vi "Control - PID Control.vi"() -> ()   [LabVIEW 2013, in "Control Workspace Object.lvlib"]
doc: "Sample numeric display item."
uses:
  Control Workspace Object.lvlib
  <vilib>/NI Veristand/Display Template Support/Display Template Support.llb/cluster_Screen Item Settings.ctl
  <vilib>/NI Veristand/Display Template Support/Display Template Support.llb/cluster_Graph Scale Settings.ctl
  <vilib>/NI Veristand/Display Template Support/Display Template Support.llb/cluster_Graph Plot Settings.ctl
  NationalInstruments.VeriStand.SystemStorage
  <vilib>/NI Veristand/Display Template Support/Display Template Support.llb/enum_Display Template Handler Minimal To Widget Msg.ctl
  <vilib>/NI Veristand/Display Template Support/Display Template Support.llb/enum_Display Template Handler Minimal To Workspace.ctl
  Shared/Types/Workspace Object State Variables.ctl
  Types/UI.Refs.ctl
  Shared/Types/UDP Streaming Command Cluster.ctl
  Shared/Types/UDP Streaming State.ctl
  Shared/Types/Workspace Object Cached Settings.ctl
  <vilib>/NI Veristand/Execution/Workspace/WorkspaceAPI.ctl
  <vilib>/NI Veristand/Execution/Workspace/SystemStateRegEventRef.ctl
  <vilib>/NI Veristand/Execution/Workspace/SystemStateEventRef.ctl
  <vilib>/NI Veristand/Display Template Support/Display Template Support.llb/sub_Display Template Handler Custom.vi
  Shared/Constants.vi
  <vilib>/NI Veristand/Execution/Workspace/NI VeriStand - Get Multiple Channel Values.vi
  <vilib>/NI Veristand/Execution/Workspace/NI VeriStand - Set Single Channel Value.vi
  Shared/Control Addon Shared.lvlib
  <vilib>/NI Veristand/Execution/Workspace/NI_VS Workspace ExecutionAPI.lvlib
  NationalInstruments.VeriStand.ClientAPI
panel:
  in  "Manual Value":bool
  in  "Revert":bool
  in  "Apply":bool
  in  "Manual Output":dbl
  in  "Manual Control":bool
  in  "Setpoint":dbl
  in  "NIVS.System Definition Root":refnum<k24>
  in  "NIVS.Gateway IP Address":string
  in  "T = PID":bool=TRUE
  in  "Hold":bool
  in  "Autoscale Y":bool=TRUE
  in  "Autoscale X":bool=TRUE
  out "Chart":waveform(dbl)[](graph)
  out "Control Name":string
  in  "Item.Data":T1
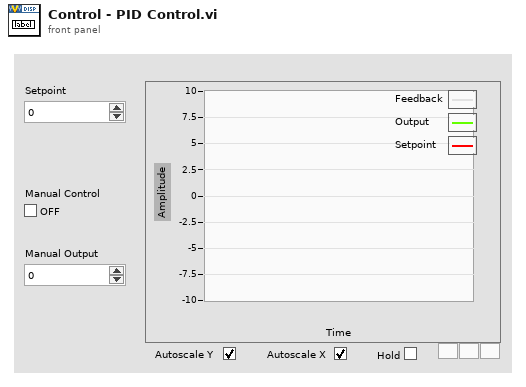
[diagram p1: front panel]
types:
  T1 = typedef "cluster_Screen Item Settings.ctl" = cluster{"Template VI":string, "Position X":i32, "Position Y":i32, "Custom":string, "Show Title Bar":bool, "ID":i32, "Always On Top":bool, "Allow Resize":bool, "Allow Minimize":bool, "Allow Close":bool, "Size to Screen":bool, "Screen.ID":i32, "State":enum16{"Normal", "New"}, "Title":string, "Window Bounds":cluster{"[0]":i16, "[1]":i16, "[2]":i16, "[3]":i16}, "Channel Ref":u64, "Unit":string, "Default Units?":bool, "Flash Limit?":bool, "Color 1":u32, "Color 2":u32, "Color 3":u32, "Color 4":u32, "Bck Color":u32, "Fore Color":u32, "Limit 1":dbl, "Limit 2":dbl, "Limit 3":dbl, "Limit 4":dbl, "Limit Mode 1":i32, "Limit Mode 2":i32, "Limit Mode 3":i32, "Limit Mode 4":i32, "Scale Precision":i32, "Scale Min":dbl, "Scale Max":dbl, "Format":i32, "Precision":i32, "Background Type":i32, "IDs":i32[], "Units":string[], "Labels":string[], "Scale Factor":dbl, "Scale Offset":dbl, "YScale Index":u32[], "XScale":T2, "YScales":T2[], "Plots":T3[], "Update Period":dbl, "History Length":dbl, "My.Ref":refnum<vi>, "Is Control?":bool, "Channel Paths":string[], "Custom Data":variant}
  T2 = typedef "cluster_Graph Scale Settings.ctl" = cluster{"Format":u8, "Precision":u8, "Fit":u8, "Label":string, "Use Default Label":bool, "Label Visible":bool, "Min":dbl, "Max":dbl}
  T3 = typedef "cluster_Graph Plot Settings.ctl" = cluster{"Bar Style":u8, "Fill To":i16, "Fill/PtColor":u32, "Line Style":u8, "Line Width":u8, "Color":u32, "Interp":u8, "Point Style":u8}
  T4 = typedef "Control Addon Shared.lvlib/Workspace Object State Variables.ctl" = cluster{"UI.Refs":T5, "Addon.GUID":string, "Addon.Name":string, "Addon.Type":enum16{"PID", "Industrial"}, "Data.UDPEngineQueue":refnum<queue>, "Data.Found?":bool, "Data.UDPChannels":string[], "Data.PreviousValues":dbl[], "Data.SlowChannels":string[], "Data.PendingChange?":bool, "CachedData.UserEvent":refnum<user-event>, "CachedData.Data":T6, "Workspace.Connected?":bool, "NIVS.SysDef":refnum<k24>, "NIVS.WorkspaceManager":T7, "NIVS.UserEventRefs":cluster{"Event Registration Refnum":refnum<event-registration>, "SystemChangeEventRef":T8}, "NIVS.SystemStateRefs":T9, "NIVS.LaunchRef":refnum<user-event>}
  T5 = typedef "Control Addon Shared.lvlib/UI.Refs.ctl" = cluster{"Chart":refnum<vi>, "Manual Value":refnum<vi>, "Manual Output":refnum<vi>, "Revert":refnum<vi>, "Apply":refnum<vi>}
  T6 = typedef "Control Addon Shared.lvlib/Workspace Object Cached Settings.ctl" = cluster{"Path":string}
  T7 = typedef "NI_VS Workspace ExecutionAPI.lvlib/WorkspaceAPI.ctl" = refnum<k24>
  T8 = typedef "NI_VS Workspace ExecutionAPI.lvlib/SystemStateRegEventRef.ctl" = refnum<event-registration>
  T9 = typedef "NI_VS Workspace ExecutionAPI.lvlib/SystemStateEventRef.ctl" = cluster{"CustDatRef":refnum<user-event>, "EvtRef":refnum<k27>}
  T10 = typedef "enum_Display Template Handler Minimal To Workspace.ctl" = cluster{"Operation":enum16{"SetCustomData", "DeleteItem"}, "Data":variant}
  T11 = typedef "enum_Display Template Handler Minimal To Widget Msg.ctl" = enum16{"Stop", "LaunchConfigDialog"}
  T12 = typedef "Control Addon Shared.lvlib/UDP Streaming Command Cluster.ctl" = cluster{"Action":T13, "Channels":string[]}
  T13 = typedef "Control Addon Shared.lvlib/UDP Streaming State.ctl" = enum8{"Idle", "Start Acq", "Run", "Stop Acq", "Exit"}
  T14 = cluster{"Event Registration Refnum":refnum<event-registration>, "SystemChangeEventRef":T8}
  T15 = typedef "NI_VS Workspace ExecutionAPI.lvlib/SystemState.ctl" = u8
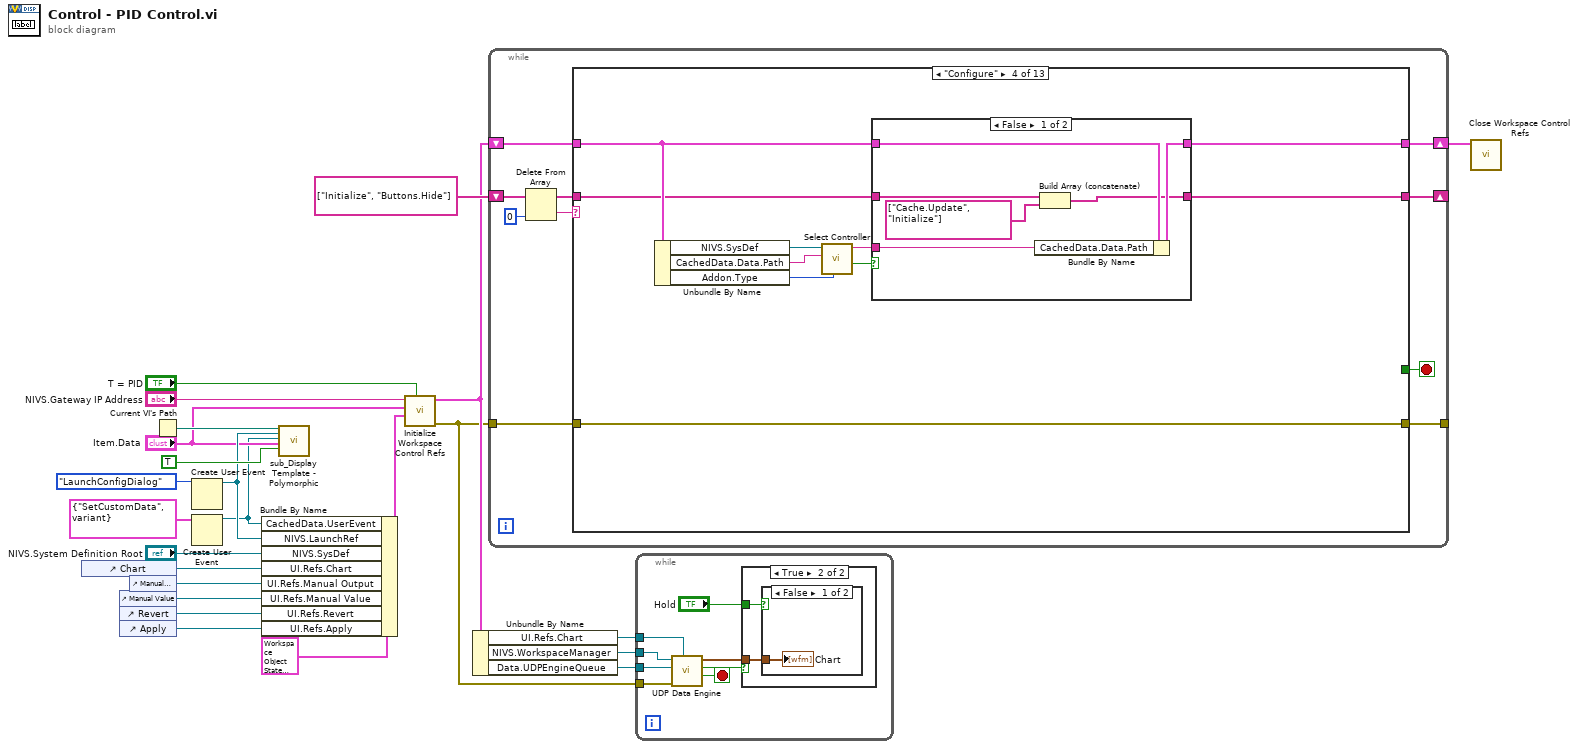
[diagram p0: block diagram]
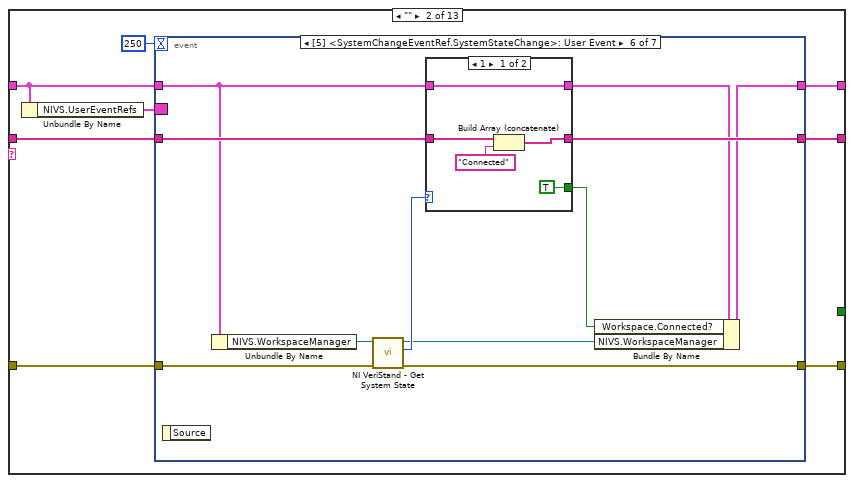
[diagram p5: hidden frame]
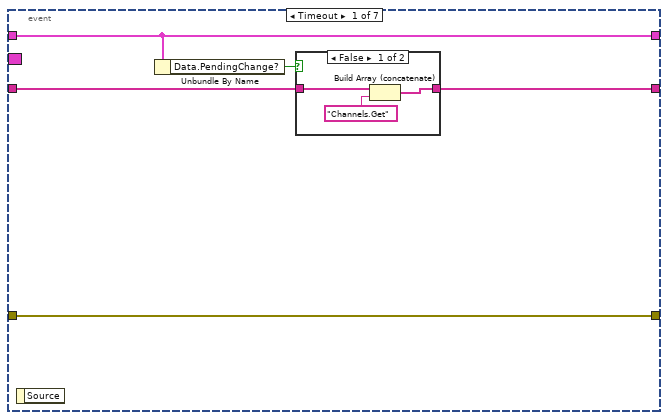
[diagram p6: hidden frame]
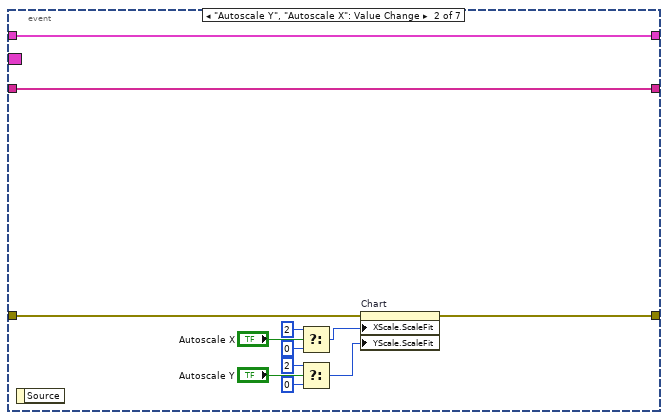
[diagram p8: hidden frame]
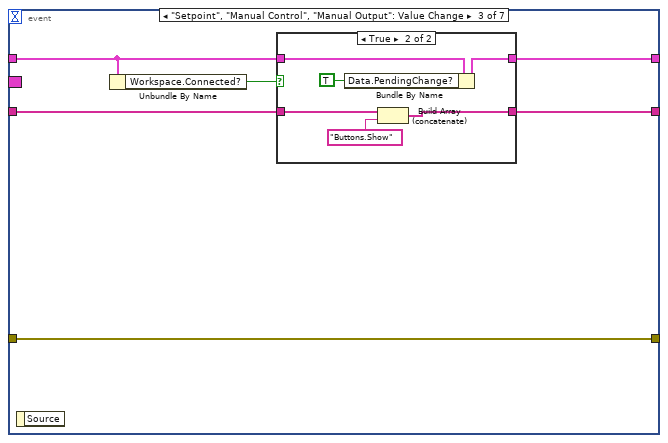
[diagram p9: hidden frame]
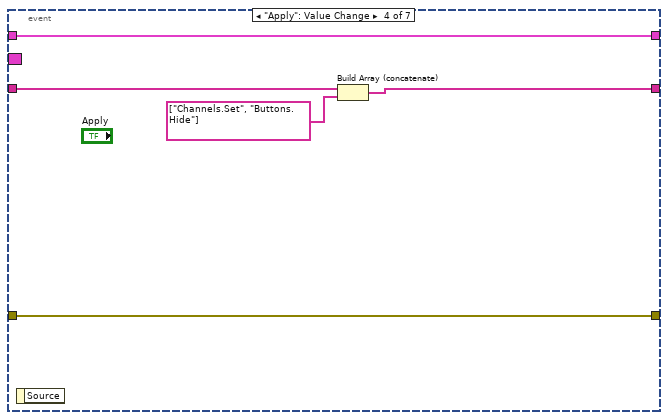
[diagram p11: hidden frame]
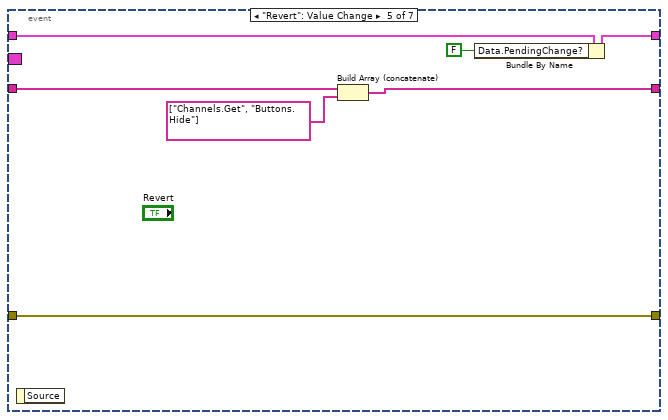
[diagram p12: hidden frame]
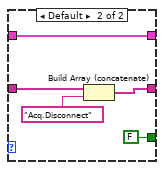
[diagram p13: hidden frame]
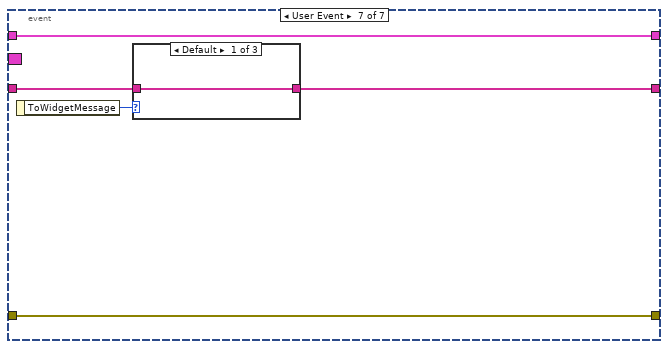
[diagram p14: hidden frame]
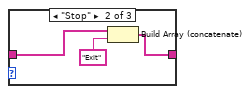
[diagram p15: hidden frame]
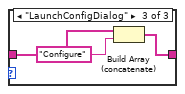
[diagram p16: hidden frame]
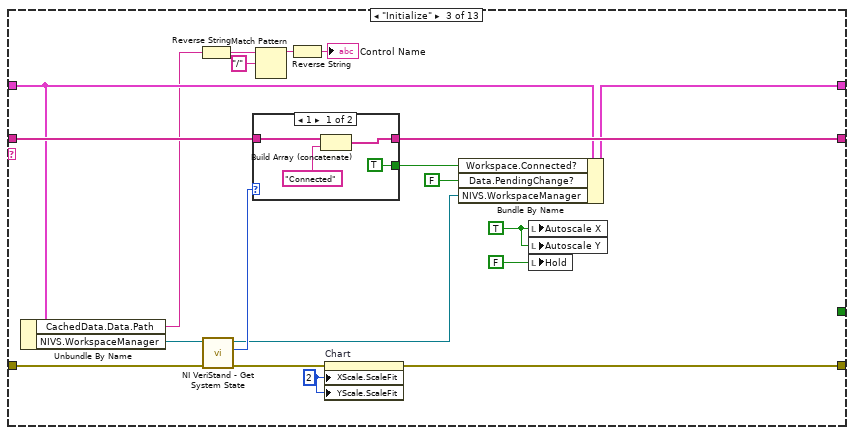
[diagram p17: hidden frame]
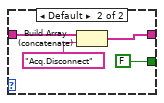
[diagram p18: hidden frame]
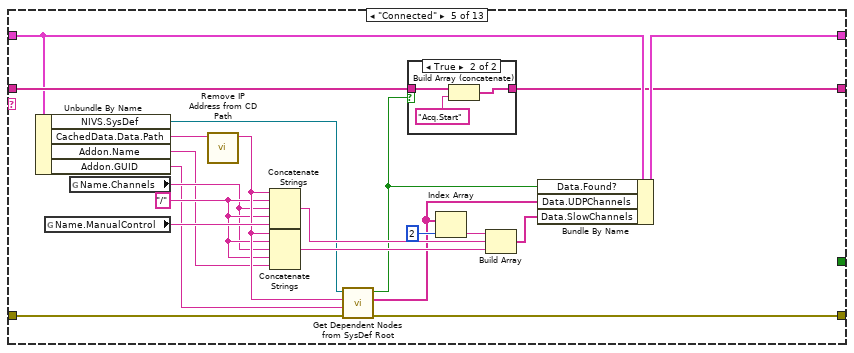
[diagram p20: hidden frame]
diagram:
  n1 = control-ref of="Chart"() -> (w12:refnum<vi>)
  n2 = control-ref of="Manual Value"() -> (w10:refnum<vi>)
  n3 = control-ref of="Revert"() -> (w9:refnum<vi>)
  n4 = control-ref of="Apply"() -> (w8:refnum<vi>)
  n5 = control-ref of="Manual Output"() -> (w11:refnum<vi>)
  n6 = Current VI's Path() -> (path=w22:path)
  n7 = Create User Event(user event datatype=enum_Display_Template_Handler_Minimal_To_Widget_Msg."LaunchConfigDialog" ("ToWidgetMessage")) -> (user event=w7:refnum<user-event>)  [unwired: 1 in, 1 out]
  n8 = Create User Event(user event datatype=T10 {"Operation"=enum."SetCustomData", "Data"=variant} ("Data")) -> (user event=w2:refnum<user-event>)  [unwired: 1 in, 1 out]
  n9 = Bundle By Name(cluster=T4 {"UI.Refs"={"Chart"=refnum, "Manual Value"=refnum, "Manual Output"=refnum, "Revert"=refnum, "Apply"=refnum}, "Addon.GUID"="", "Addon.Name"="", "Addon.Type"=enum."PID", "Data.UDPEngineQueue"=refnum, "Data.Found?"=FALSE, "Data.UDPChannels"=[], "Data.PreviousValues"=[], "Data.SlowChannels"=[], "Data.PendingChange?"=FALSE, "CachedData.UserEvent"=refnum, "CachedData.Data"={"Path"=""}, "Workspace.Connected?"=FALSE, "NIVS.SysDef"=refnum, "NIVS.WorkspaceManager"=refnum, "NIVS.UserEventRefs"={"Event Registration Refnum"=refnum, "SystemChangeEventRef"=refnum}, "NIVS.SystemStateRefs"={"CustDatRef"=refnum, "EvtRef"=refnum}, "NIVS.LaunchRef"=refnum}, "CachedData.UserEvent"=w2, "NIVS.LaunchRef"=w7, "NIVS.SysDef"="NIVS.System Definition Root", "UI.Refs.Chart"=w12, "UI.Refs.Manual Output"=w11, "UI.Refs.Manual Value"=w10, "UI.Refs.Revert"=w9, "UI.Refs.Apply"=w8) -> (w4:T4)
  n10 = call-poly <vilib>:"sub_Display Template - Polymorphic.vi"("Parent.Path"=w22, "ToWidgetEvent"=w7, "ToWorkspace"=w2, "Item.Data"="Item.Data", "Resizable"=TRUE) -> ()  [unwired: 1 in, 14 out]
  n11 = call "Initialize Workspace Control Refs.vi"("T = PID"="T = PID", "State Variables in"=w4, "Item.Data"="Item.Data", "NIVS.Gateway IP Address"="NIVS.Gateway IP Address") -> ("error out"=w1:errorcluster, "State Variables out"=w15:T4)  [unwired: 6 in]
  n12 = Unbundle By Name(w15) -> ("UI.Refs.Chart"=w17:refnum<vi>, "NIVS.WorkspaceManager"=w16:T7, "Data.UDPEngineQueue"=w14:refnum<queue>)
  n13 = while {
    shift-right: [w28] -> _
    shift-left: string[] ["Initialize", "Buttons.Hide"] -> [w32]
    tunnel: w1 -> [w30]
    tunnel: [w27] -> _
    shift-right: [w26] -> w19
    shift-left: w15 -> [w25]
    stop <- w34 stop-if-true
    n14 = Delete From Array(array=w32, index=0) -> (deleted portion=w31:string, array with subset deleted=w29:string[])  [unwired: 1 in]
    n15 = case shown="\"Configure\"" w31 {
      tunnel: [_ _ _ _ _ TRUE _ _ _ _ _ _ _] -> w34
      tunnel: [w37 w44 w142 w157 w181 w206 w213 w221 w229 w235 w241 w252 w304] -> w28
      tunnel: w30 -> [w36 w42 w144 w163 w173 w201 w212 w216 w228 w231 w237 w249 w292]
      tunnel: w29 -> [w37 w43 w143 w156 w192 w206 w213 w221 w229 w235 w241 w252 w304]
      tunnel: w25 -> [w35 w38 w130 w161 w190 w198 w209 w220 w224 w234 w240 w242 w290]
      tunnel: [w36 w41 w126 w163 w191 w200 w212 w215 w227 w230 w236 w248 w291] -> w27
      tunnel: [w35 w40 w137 w160 w189 w198 w209 w220 w224 w234 w240 w247 w289] -> w26
      frame Default {
      }
      frame "" {
        n16 = Unbundle By Name(w38) -> ("NIVS.UserEventRefs"=w39:T14)
        n17 = event shown="[5] <SystemChangeEventRef.SystemStateChange>: User Event" {
          selector: w39 -> [_ _ _ _ _ _ _]
          dyn-events: _ -> [_ _ _ _ _ _ _]
          timeout: 250 -> [_ _ _ _ _ _ _]
          tunnel: [w48 w66 w69 w81 w89 w99 w117] -> w44
          tunnel: w43 -> [w49 w66 w70 w82 w90 w100 w116]
          tunnel: w42 -> [w50 w60 w72 w85 w92 w103 w115]
          tunnel: [w50 w59 w72 w85 w92 w102 w115] -> w41
          tunnel: [w47 w65 w71 w84 w87 w98 w114] -> w40
          tunnel: w38 -> [w47 w65 w68 w84 w88 w95 w114]
          event Timeout {
            n18 = event-data() -> ()  [unwired: 2 out]
            n19 = Unbundle By Name(w47) -> ("Data.PendingChange?"=w46:bool)
            n20 = case shown="False" w46 {
              tunnel: w49 -> [w52 w54]
              tunnel: [w51 w54] -> w48
              frame False {
                n21 = Build Array (concatenate)(w52, "Channels.Get") -> (w51:string[])
              }
              frame True {
              }
            }
          }
          event "Autoscale Y", "Autoscale X": Value Change {
            n22 = event-data() -> ()  [unwired: 2 out]
            n23 = Select(t=u8 2, s="Autoscale X", f=u8 0 ("X Scale.Scale Fit")) -> (s? t:f=w62:u8)
            n24 = Select(t=u8 2, s="Autoscale Y", f=u8 0 ("X Scale.Scale Fit")) -> (s? t:f=w55:u8)
            n25 = property on="Chart" class="WFChart (strict)"(error in=w60, "XScale.ScaleFit"=w62, "YScale.ScaleFit"=w55) -> (error out=w59:errorcluster)  [unwired: 1 in, 1 out]
          }
          event "Setpoint", "Manual Control", "Manual Output": Value Change {
            n26 = event-data() -> ()  [unwired: 2 out]
            n27 = Unbundle By Name(w68) -> ("Workspace.Connected?"=w67:bool)
            n28 = case shown="True" w67 {
              tunnel: w68 -> [w73 w79]
              tunnel: [w73 w78] -> w71
              tunnel: w70 -> [w74 w77]
              tunnel: [w74 w75] -> w69
              frame False {
              }
              frame True {
                n29 = Bundle By Name(cluster=w79, "Data.PendingChange?"=TRUE ("Pending Change?")) -> (w78:T4)
                n30 = Build Array (concatenate)(w77, "Buttons.Show") -> (w75:string[])
              }
            }
          }
          event "Apply": Value Change {
            n31 = event-data() -> ()  [unwired: 2 out]
            n32 = Build Array (concatenate)(w82, string[] ["Channels.Set", "Buttons.Hide"]) -> (w81:string[])
          }
          event "Revert": Value Change {
            n33 = event-data() -> ()  [unwired: 2 out]
            n34 = Build Array (concatenate)(w90, string[] ["Channels.Get", "Buttons.Hide"]) -> (w89:string[])
            n35 = Bundle By Name(cluster=w88, "Data.PendingChange?"=FALSE ("Pending Change?")) -> (w87:T4)
          }
          event User Event {
            n36 = event-data() -> ()  [unwired: 2 out]
            n37 = Unbundle By Name(w95) -> ("NIVS.WorkspaceManager"=w94:T7)
            n38 = call <vilib>:"NI VeriStand - Get System State.vi"("error in (no error)"=w103, "WorkspaceManager in"=w94) -> ("error out"=w102:errorcluster, "System State"=w101:T15, "WorkspaceManager  out"=w93:T7)  [unwired: 5 in, 2 out]
            n39 = case shown="1" w101 {
              tunnel: w100 -> [w108 w113]
              tunnel: [w107 w112] -> w99
              tunnel: [w105 w110] -> w97
              tunnel: w95 -> [w105 w110]
              tunnel: [TRUE FALSE] -> w96
              frame 1 {
                n40 = Build Array (concatenate)(w108, "Connected") -> (w107:string[])
              }
              frame Default {
                n41 = Build Array (concatenate)(w113, "Acq.Disconnect") -> (w112:string[])
              }
            }
            n42 = Bundle By Name(cluster=w97, "Workspace.Connected?"=w96, "NIVS.WorkspaceManager"=w93) -> (w98:T4)
          }
          event User Event {
            n43 = event-data() -> ("ToWidgetMessage"=w118:T11)  [unwired: 1 out]
            n44 = case shown="Default" w118 {
              tunnel: [w119 w121 w124] -> w117
              tunnel: w116 -> [w119 w122 w125]
              frame Default {
              }
              frame "Stop" {
                n45 = Build Array (concatenate)(w122, "Exit") -> (w121:string[])
              }
              frame "LaunchConfigDialog" {
                n46 = Build Array (concatenate)(w125, "Configure") -> (w124:string[])
              }
            }
          }
        }
      }
      frame "Initialize" {
        w134 = u8 2 ("X Scale.Scale Fit")
        w135 = TRUE ("Autoscale X")
        n47 = Unbundle By Name(w130) -> ("CachedData.Data.Path"=w128:string, "NIVS.WorkspaceManager"=w129:T7)
        n48 = Reverse String(1:w128) -> (0:w141:string)
        n49 = call <vilib>:"NI VeriStand - Get System State.vi"("error in (no error)"=w144, "WorkspaceManager in"=w129) -> ("error out"=w133:errorcluster, "System State"=w145:T15, "WorkspaceManager  out"=w127:T7)  [unwired: 5 in, 2 out]
        n50 = case shown="1" w145 {
          tunnel: w143 -> [w149 w153]
          tunnel: [w148 w152] -> w142
          tunnel: [TRUE FALSE] -> w136
          frame 1 {
            n51 = Build Array (concatenate)(w149, "Connected") -> (w148:string[])
          }
          frame Default {
            n52 = Build Array (concatenate)(w153, "Acq.Disconnect") -> (w152:string[])
          }
        }
        n53 = Match Pattern(string=w141, regular expression="/") -> (before substring=w138:string)  [unwired: 1 in, 3 out]
        n54 = Reverse String(1:w138) -> (0:→"Control Name":string)
        n55 = property on="Chart" class="WFChart (strict)"(error in=w133, "XScale.ScaleFit"=w134, "YScale.ScaleFit"=w134) -> (error out=w126:errorcluster)  [unwired: 1 in, 1 out]
        n56 = Bundle By Name(cluster=w130, "Workspace.Connected?"=w136, "Data.PendingChange?"=FALSE ("Pending Change?"), "NIVS.WorkspaceManager"=w127) -> (w137:T4)
        n57 = local write "Autoscale X"(w135) -> ()
        n58 = local write "Autoscale Y"(w135) -> ()
        n59 = local write "Hold"(FALSE ("Hold")) -> ()
      }
      frame "Configure" {
        n60 = Unbundle By Name(w161) -> ("NIVS.SysDef"=w155:refnum<k24>, "CachedData.Data.Path"=w162:string, "Addon.Type"=w154:enum16{"PID", "Industrial"})
        n61 = call "Select Controller.vi"("Type"=w154, "CD Path"=w162, "NIVS.System Definition Root"=w155) -> ("Cancelled?"=w159:bool, "Custom Device Path Out"=w158:string)  [unwired: 6 in, 1 out]
        n62 = case shown="False" w159 {
          tunnel: w161 -> [w169 w170]
          tunnel: [w168 w170] -> w160
          tunnel: w158 -> [w167 _]
          tunnel: [w165 w171] -> w157
          tunnel: w156 -> [w166 w171]
          frame False {
            n63 = Bundle By Name(cluster=w169, "CachedData.Data.Path"=w167) -> (w168:T4)
            n64 = Build Array (concatenate)(w166, string[] ["Cache.Update", "Initialize"]) -> (w165:string[])
          }
          frame True {
          }
        }
      }
      frame "Connected" {
        w178 = "/" ("string")
        n65 = Unbundle By Name(w190) -> ("NIVS.SysDef"=w174:refnum<k24>, "CachedData.Data.Path"=w188:string, "Addon.Name"=w175:string, "Addon.GUID"=w172:string)
        n66 = global read "Constants.vi" "Name.ManualControl"() -> (w187:string)
        n67 = global read "Constants.vi" "Name.Channels"() -> (w177:string)
        n68 = call "Remove IP Address from CD Path.vi"("CD Path"=w188) -> ("Path"=w186:string)  [unwired: 10 in]
        n69 = Concatenate Strings(w186, w178, w177, w178, w187) -> (w185:string)
        n70 = Concatenate Strings(w186, w178, w177, w178, w175) -> (w184:string)
        n71 = call "Get Dependent Nodes from SysDef Root.vi"("error in (no error)"=w173, "GUID"=w172, "Path"=w186, "SysDef Ref"=w174) -> ("error out"=w191:errorcluster, "Channels"=w180:string[], "Found"=w176:bool)  [unwired: 5 in]
        n72 = case shown="True" w176 {
          tunnel: w192 -> [w193 w196]
          tunnel: [w193 w195] -> w181
          frame False {
          }
          frame True {
            n73 = Build Array (concatenate)(w196, "Acq.Start") -> (w195:string[])
          }
        }
        n74 = Index Array(array=w180, index=2) -> (element=w182:string)
        n75 = Build Array(w182, w185, w184) -> (w179:string[])
        n76 = Bundle By Name(cluster=w190, "Data.Found?"=w176, "Data.UDPChannels"=w180, "Data.SlowChannels"=w179) -> (w189:T4)
      }
      frame "Exit" {
        n77 = Unbundle By Name(w198) -> ("Data.UDPEngineQueue"=w197:refnum<queue>)
        n78 = Enqueue Element(queue=w197, element=T12 {"Action"=enum."Stop Acq", "Channels"=[]}, error in (no error)=w201) -> (queue out=w204:refnum<queue>, error out=w202:errorcluster)  [unwired: 1 in, 1 out]
        n79 = Enqueue Element(queue=w204, element=T12 {"Action"=enum."Exit", "Channels"=[]}, error in (no error)=w202) -> (error out=w200:errorcluster)  [unwired: 1 in, 2 out]
      }
      frame "Cache.Update" {
        n80 = Unbundle By Name(w209) -> ("CachedData.UserEvent"=w207:refnum<user-event>, "CachedData.Data"=w208:T6)
        n81 = Bundle By Name(cluster=T10 {"Operation"=enum."SetCustomData", "Data"=variant} ("event data"), "Data"=w208) -> (w210:T10)
        n82 = Generate User Event(user event=w207, event data cluster=w210) -> ()  [unwired: 2 in, 2 out]
      }
      frame "Acq.Start" {
        n83 = Unbundle By Name(w220) -> ("Data.UDPEngineQueue"=w214:refnum<queue>, "Data.UDPChannels"=w218:string[])
        n84 = Bundle By Name(cluster=T12 {"Action"=enum."Start Acq", "Channels"=[]}, "Channels"=w218) -> (w217:T12)
        n85 = Enqueue Element(queue=w214, element=w217, error in (no error)=w216) -> (error out=w215:errorcluster)  [unwired: 1 in, 2 out]
      }
      frame "Acq.Disconnect" {
        w222 = FALSE ("Manual Control")
        w225 = 0.0 ("Setpoint")
        n86 = Unbundle By Name(w224) -> ("Data.UDPEngineQueue"=w223:refnum<queue>)
        n87 = Enqueue Element(queue=w223, element=T12 {"Action"=enum."Stop Acq", "Channels"=[]}, error in (no error)=w228) -> (error out=w227:errorcluster)  [unwired: 1 in, 2 out]
        n88 = local write "Setpoint"(w225) -> ()
        n89 = local write "Manual Output"(w225) -> ()
        n90 = local write "Manual Control"(w222) -> ()
        n91 = local write "Manual Value"(w222) -> ()
      }
      frame "Buttons.Hide" {
        w232 = FALSE ("Hold")
        n92 = property on="Apply" class="Bool"(error in=w231, "Visible"=w232) -> (error out=w233:errorcluster)  [unwired: 1 in, 1 out]
        n93 = property on="Revert" class="Bool"(error in=w233, "Visible"=w232) -> (error out=w230:errorcluster)  [unwired: 1 in, 1 out]
      }
      frame "Buttons.Show" {
        w238 = TRUE ("Hold")
        n94 = property on="Apply" class="Bool"(error in=w237, "Visible"=w238) -> (error out=w239:errorcluster)  [unwired: 1 in, 1 out]
        n95 = property on="Revert" class="Bool"(error in=w239, "Visible"=w238) -> (error out=w236:errorcluster)  [unwired: 1 in, 1 out]
      }
      frame "Channels.Get" {
        n96 = Unbundle By Name(w242) -> ("Data.PendingChange?"=w243:bool, "Addon.Type"=w246:enum16{"PID", "Industrial"}, "Data.Found?"=w250:bool, "Workspace.Connected?"=w251:bool, "NIVS.WorkspaceManager"=w245:T7, "Data.SlowChannels"=w244:string[])
        n97 = case shown="False" w243 {
          tunnel: w251 -> [w269 _]
          tunnel: w250 -> [w263 _]
          tunnel: w249 -> [w260 w283]
          tunnel: [w259 w283] -> w248
          tunnel: [w258 w284] -> w247
          tunnel: w246 -> [w257 _]
          tunnel: w245 -> [w256 _]
          tunnel: w244 -> [w254 _]
          tunnel: w242 -> [w253 w284]
          frame False {
            n98 = Compound Arithmetic op=AND(w263, w269) -> (w264:bool)
            n99 = case shown="True" w264 {
              tunnel: w260 -> [w276 w282]
              tunnel: [w276 w281] -> w259
              tunnel: w256 -> [w275 w280]
              tunnel: [w275 w279] -> w255
              tunnel: w254 -> [_ w278]
              tunnel: [dbl[] [0.0, 0.0, 0.0] ("Values") w277] -> w268
              frame False {
              }
              frame True {
                n100 = call-poly <vilib>:"NI VeriStand - Get Channel Value.vi"("error in (no error)"=w282, "Channels"=w278, "WorkspaceManager in"=w280) -> ("error out"=w281:errorcluster, "Values"=w277:dbl[], "WorkspaceManager out"=w279:T7)  [unwired: 6 in]
              }
            }
            n101 = Index Array(array=w268) -> (element #1=w267:dbl, element #2=w262:dbl, element #3=w261:dbl)  [unwired: 3 in]
            n102 = To Long Integer(number=w262) -> (32bit integer=w266:i32)
            n103 = case shown="\"Industrial\"" w257 {
              tunnel: w261 -> [w271 w273]
              frame "Industrial" {
                n104 = To Long Integer(number=w271) -> (32bit integer=w272:i32)
                n105 = Not Equal To 0?(x=w272) -> (x != 0?=w270:bool)
                n106 = local write "Manual Value"(w270) -> ()
              }
              frame "PID" {
                n107 = local write "Manual Output"(w273) -> ()
              }
            }
            n108 = Not Equal To 0?(x=w266) -> (x != 0?=w265:bool)
            n109 = local write "Setpoint"(w267) -> ()
            n110 = local write "Manual Control"(w265) -> ()
            n111 = Bundle By Name(cluster=w253, "NIVS.WorkspaceManager"=w255, "Data.PreviousValues"=w268) -> (w258:T4)
          }
          frame True {
          }
        }
      }
      frame "Channels.Set" {
        n112 = Unbundle By Name(w290) -> ("Data.Found?"=w295:bool, "Workspace.Connected?"=w298:bool, "Data.PreviousValues"=w297:dbl[], "Data.SlowChannels"=w299:string[], "NIVS.WorkspaceManager"=w287:T7, "Addon.Type"=w285:enum16{"PID", "Industrial"})
        n113 = case shown="\"Industrial\"" w285 {
          tunnel: [w306 "Manual Output"] -> w293
          frame "Industrial" {
            n114 = Boolean To (0,1)(Boolean="Manual Value") -> (0, 1=w306:i16)
          }
          frame "PID" {
          }
        }
        n115 = Boolean To (0,1)(Boolean="Manual Control") -> (0, 1=w294:i16)
        n116 = Build Array("Setpoint", w294, w293) -> (w300:dbl[])
        n117 = Not Equal?(x=w297, y=w300) -> (x != y?=w303:bool[])
        n118 = Compound Arithmetic op=AND(w295, w298) -> (w296:bool)
        n119 = case shown="True" w296 {
          tunnel: w303 -> [_ w316]
          tunnel: w300 -> [_ w315]
          tunnel: w292 -> [w309 w314]
          tunnel: [w309 w313] -> w291
          tunnel: w287 -> [w308 w312]
          tunnel: [w308 w311] -> w286
          tunnel: w299 -> [_ w310]
          frame False {
          }
          frame True {
            n120 = for {
              shift-right: [w322] -> w313
              shift-left: w314 -> [w323]
              shift-right: [w321] -> w311
              shift-left: w312 -> [w320]
              tunnel: w316 -> [w319] mode=indexing
              tunnel: w315 -> [w318] mode=indexing
              tunnel: w310 -> [w317] mode=indexing
              n121 = case shown="True" w319 {
                tunnel: w323 -> [w325 w331]
                tunnel: [w325 w330] -> w322
                tunnel: [w324 w329] -> w321
                tunnel: w320 -> [w324 w328]
                tunnel: w318 -> [_ w327]
                tunnel: w317 -> [_ w326]
                frame False {
                }
                frame True {
                  n122 = call-poly <vilib>:"NI VeriStand - Set Channel Value.vi"("error in (no error)"=w331, "Value"=w327, "Channel"=w326, "WorkspaceManager in"=w328) -> ("error out"=w330:errorcluster, "WorkspaceManager out"=w329:T7)  [unwired: 6 in]
                }
              }
            }
          }
        }
        n123 = Bundle By Name(cluster=w290, "Data.PendingChange?"=FALSE ("Pending Change?"), "NIVS.WorkspaceManager"=w286) -> (w289:T4)
      }
    }
  }
  n124 = while {
    tunnel: w16 -> [w334]
    tunnel: w14 -> [w339]
    tunnel: w17 -> [w335]
    tunnel: w1 -> [w333]
    stop <- w338 stop-if-true
    n125 = call "UDP Data Engine.vi"("WaveformChart Ref"=w335, "error in (no error)"=w333, "UDP Engine Queue"=w339, "WorkspaceManager"=w334) -> ("Exit"=w338:bool, "Update?"=w332:bool, "Waveform"=w336:waveform(dbl)[])  [unwired: 4 in, 1 out]
    n126 = case shown="True" w332 {
      tunnel: "Hold" -> [_ w341]
      tunnel: w336 -> [_ w340]
      frame False {
      }
      frame True {
        n127 = case shown="False" w341 {
          tunnel: w340 -> [w342 _]
          frame False {
            "Chart" <- w342
          }
          frame True {
          }
        }
      }
    }
  }
  n128 = call "Close Workspace Control Refs.vi"("State Variables in"=w19) -> ()  [unwired: 11 in]
